vi "Untitled 1.vi"() -> ()   [LabVIEW 2012]
uses:
  Control 1.ctl
panel:
  out "Boolean":bool
  in  "OK Button 7":bool
  in  "CE":bool
  in  "MC":bool
  in  "MR":bool
  in  "MS":bool
  in  "x^2":bool
  in  "1/x":bool
  in  "sqrt":bool
  in  "+/-":bool
  in  "-":bool
  in  "x":bool
  in  "/":bool
  in  "C":bool
  in  ",":bool
  in  "0":bool
  in  "9":bool
  in  "8":bool
  in  "7":bool
  in  "6":bool
  in  "5":bool
  in  "4":bool
  in  "3":bool
  out "екран":string
  in  "=":bool
  in  "+":bool
  in  "2":bool
  in  "1":bool
  in  "stop":bool
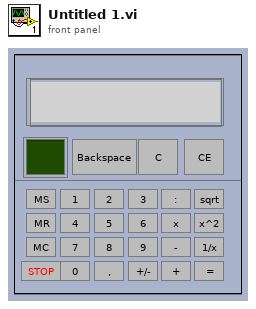
[diagram p1: front panel]
types:
  T1 = typedef "Control 1.ctl" = enum16{"mc", "mr", "ms", "ce", "c", "1/x", "x^2", "sqrt", "+/-", "m", "x", "/", ",", "4", "5", "6", "7", "8", "9", "0", "3", "event", "стоп", "1", "2", "+", "="}
  T2 = cluster{"екран":string, "чистий екран":string, "буфер":string, "Enum":T1, "ms":string, "mr":string}
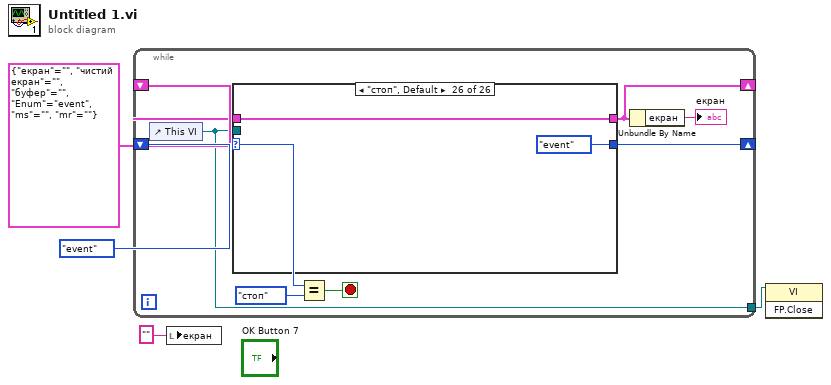
[diagram p0: block diagram]
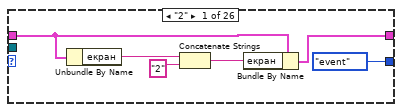
[diagram p2: hidden frame]
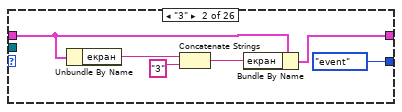
[diagram p3: hidden frame]
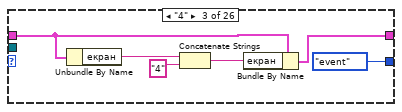
[diagram p4: hidden frame]
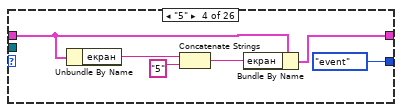
[diagram p5: hidden frame]
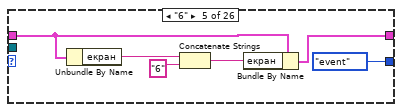
[diagram p6: hidden frame]
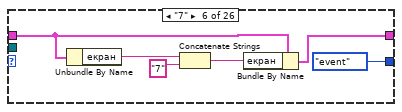
[diagram p7: hidden frame]
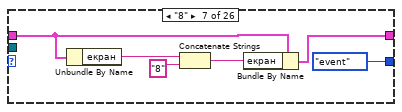
[diagram p8: hidden frame]
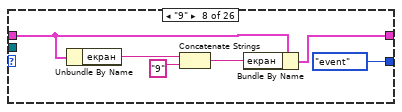
[diagram p9: hidden frame]
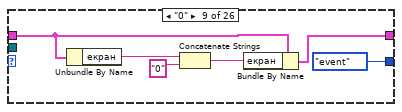
[diagram p10: hidden frame]
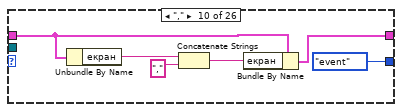
[diagram p11: hidden frame]
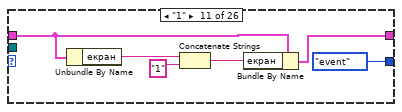
[diagram p12: hidden frame]
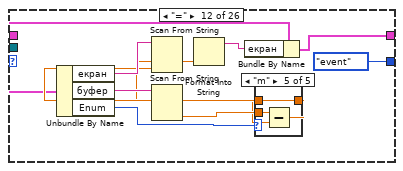
[diagram p13: hidden frame]
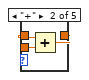
[diagram p15: hidden frame]
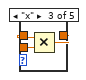
[diagram p16: hidden frame]
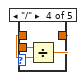
[diagram p17: hidden frame]
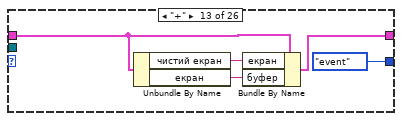
[diagram p18: hidden frame]
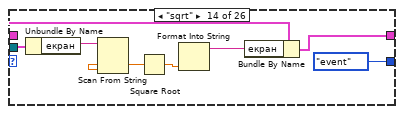
[diagram p19: hidden frame]
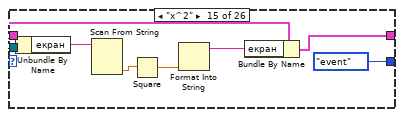
[diagram p20: hidden frame]
diagram:
  n1 = while {
    shift-right: [w12] -> _
    shift-left: Control_1."event" ("Enum") -> [w6]
    shift-right: [w8] -> _
    shift-left: T2 {"екран"="", "чистий екран"="", "буфер"="", "Enum"=enum."event", "ms"="", "mr"=""} -> [w9]
    tunnel: [w5] -> w1
    stop <- w10 stop-if-true
    n2 = control-ref of="This VI"() -> (w5:refnum<vi>)
    n3 = case shown="\"стоп\", Default" w6 {
      tunnel: [Control_1."event" ("Enum") Control_1."event" ("Enum") Control_1."event" ("Enum") Control_1."event" ("Enum") Control_1."event" ("Enum") Control_1."event" ("Enum") Control_1."event" ("Enum") Control_1."event" ("Enum") Control_1."event" ("Enum") Control_1."event" ("Enum") Control_1."event" ("Enum") Control_1."event" ("Enum") Control_1."event" ("Enum") Control_1."event" ("Enum") Control_1."event" ("Enum") Control_1."event" ("Enum") Control_1."event" ("Enum") Control_1."event" ("Enum") Control_1."event" ("Enum") w145 Control_1."event" ("Enum") Control_1."event" ("Enum") Control_1."event" ("Enum") Control_1."event" ("Enum") Control_1."event" ("Enum") Control_1."event" ("Enum")] -> w12
      tunnel: w9 -> [w17 w23 w29 w35 w41 w47 w53 w59 w65 w71 w75 w81 w105 w113 w120 w127 w131 w136 w141 w144 w246 w251 w255 w260 w264 w265]
      tunnel: [w16 w22 w28 w34 w40 w46 w52 w58 w64 w70 w74 w79 w104 w112 w119 w126 w130 w135 w140 w143 _ w250 w252 w258 w261 w265] -> w8
      tunnel: w5 -> [_ _ _ _ _ _ _ _ _ _ _ _ _ _ _ _ _ _ _ _ _ _ _ _ _ _]
      frame "2" {
        n4 = Unbundle By Name(w17) -> ("екран"=w15:string)
        n5 = Concatenate Strings(w15, "2" ("string")) -> (w13:string)
        n6 = Bundle By Name(cluster=w17, "екран"=w13) -> (w16:T2)
      }
      frame "3" {
        n7 = Unbundle By Name(w23) -> ("екран"=w21:string)
        n8 = Concatenate Strings(w21, "3" ("string")) -> (w19:string)
        n9 = Bundle By Name(cluster=w23, "екран"=w19) -> (w22:T2)
      }
      frame "4" {
        n10 = Unbundle By Name(w29) -> ("екран"=w27:string)
        n11 = Concatenate Strings(w27, "4" ("string")) -> (w25:string)
        n12 = Bundle By Name(cluster=w29, "екран"=w25) -> (w28:T2)
      }
      frame "5" {
        n13 = Unbundle By Name(w35) -> ("екран"=w33:string)
        n14 = Concatenate Strings(w33, "5" ("string")) -> (w31:string)
        n15 = Bundle By Name(cluster=w35, "екран"=w31) -> (w34:T2)
      }
      frame "6" {
        n16 = Unbundle By Name(w41) -> ("екран"=w39:string)
        n17 = Concatenate Strings(w39, "6" ("string")) -> (w37:string)
        n18 = Bundle By Name(cluster=w41, "екран"=w37) -> (w40:T2)
      }
      frame "7" {
        n19 = Unbundle By Name(w47) -> ("екран"=w45:string)
        n20 = Concatenate Strings(w45, "7" ("string")) -> (w43:string)
        n21 = Bundle By Name(cluster=w47, "екран"=w43) -> (w46:T2)
      }
      frame "8" {
        n22 = Unbundle By Name(w53) -> ("екран"=w51:string)
        n23 = Concatenate Strings(w51, "8" ("string")) -> (w49:string)
        n24 = Bundle By Name(cluster=w53, "екран"=w49) -> (w52:T2)
      }
      frame "9" {
        n25 = Unbundle By Name(w59) -> ("екран"=w57:string)
        n26 = Concatenate Strings(w57, "9" ("string")) -> (w55:string)
        n27 = Bundle By Name(cluster=w59, "екран"=w55) -> (w58:T2)
      }
      frame "0" {
        n28 = Unbundle By Name(w65) -> ("екран"=w63:string)
        n29 = Concatenate Strings(w63, "0" ("string")) -> (w61:string)
        n30 = Bundle By Name(cluster=w65, "екран"=w61) -> (w64:T2)
      }
      frame "," {
        n31 = Unbundle By Name(w71) -> ("екран"=w69:string)
        n32 = Concatenate Strings(w69, "," ("string")) -> (w67:string)
        n33 = Bundle By Name(cluster=w71, "екран"=w67) -> (w70:T2)
      }
      frame "1" {
        n34 = Unbundle By Name(w75) -> ("екран"=w77:string)
        n35 = Concatenate Strings(w77, "1" ("string")) -> (w73:string)
        n36 = Bundle By Name(cluster=w75, "екран"=w73) -> (w74:T2)
      }
      frame "=" {
        n37 = Unbundle By Name(w81) -> ("екран"=w86:string, "буфер"=w84:string, "Enum"=w87:T1)
        n38 = Scan From String(input string=w86) -> (output 1=w85:dbl)  [unwired: 4 in, 3 out]
        n39 = Scan From String(input string=w84) -> (output 1=w83:dbl)  [unwired: 4 in, 3 out]
        n40 = case shown="\"m\"" w87 {
          tunnel: w85 -> [w89 w92 w94 w97 w99]
          tunnel: w83 -> [_ w91 w95 w96 w100]
          tunnel: [w89 w90 w93 w98 w101] -> w82
          frame "event", Default {
          }
          frame "+" {
            n41 = Add(x=w92, y=w91) -> (x+y=w90:dbl)
          }
          frame "x" {
            n42 = Multiply(x=w94, y=w95) -> (x*y=w93:dbl)
          }
          frame "/" {
            n43 = Divide(x=w96, y=w97) -> (x/y=w98:dbl)
          }
          frame "m" {
            n44 = Subtract(x=w100, y=w99) -> (x-y=w101:dbl)
          }
        }
        n45 = Format Into String(w82) -> (resulting string=w80:string)  [unwired: 3 in, 1 out]
        n46 = Bundle By Name(cluster=w81, "екран"=w80) -> (w79:T2)
      }
      frame "+" {
        n47 = Unbundle By Name(w105) -> ("чистий екран"=w103:string, "екран"=w102:string)
        n48 = Bundle By Name(cluster=w105, "екран"=w103, "буфер"=w102) -> (w104:T2)
      }
      frame "sqrt" {
        n49 = Unbundle By Name(w113) -> ("екран"=w111:string)
        n50 = Scan From String(input string=w111) -> (output 1=w110:dbl)  [unwired: 4 in, 3 out]
        n51 = Square Root(x=w110) -> (sqrt(x)=w109:dbl)
        n52 = Format Into String(w109) -> (resulting string=w108:string)  [unwired: 3 in, 1 out]
        n53 = Bundle By Name(cluster=w113, "екран"=w108) -> (w112:T2)
      }
      frame "x^2" {
        n54 = Unbundle By Name(w120) -> ("екран"=w118:string)
        n55 = Scan From String(input string=w118) -> (output 1=w116:dbl)  [unwired: 4 in, 3 out]
        n56 = Square(x=w116) -> (x^2=w115:dbl)
        n57 = Format Into String(w115) -> (resulting string=w117:string)  [unwired: 3 in, 1 out]
        n58 = Bundle By Name(cluster=w120, "екран"=w117) -> (w119:T2)
      }
      frame "1/x" {
        n59 = Unbundle By Name(w127) -> ("екран"=w124:string)
        n60 = Scan From String(input string=w124) -> (output 1=w123:dbl)  [unwired: 4 in, 3 out]
        n61 = Reciprocal(x=w123) -> (1/x=w122:dbl)
        n62 = Format Into String(w122) -> (resulting string=w125:string)  [unwired: 3 in, 1 out]
        n63 = Bundle By Name(cluster=w127, "екран"=w125) -> (w126:T2)
      }
      frame "/" {
        n64 = Unbundle By Name(w131) -> ("чистий екран"=w129:string, "екран"=w128:string)
        n65 = Bundle By Name(cluster=w131, "екран"=w129, "буфер"=w128) -> (w130:T2)
      }
      frame "m" {
        n66 = Unbundle By Name(w136) -> ("чистий екран"=w134:string, "екран"=w133:string)
        n67 = Bundle By Name(cluster=w136, "екран"=w134, "буфер"=w133) -> (w135:T2)
      }
      frame "x" {
        n68 = Unbundle By Name(w141) -> ("чистий екран"=w139:string, "екран"=w138:string)
        n69 = Bundle By Name(cluster=w141, "екран"=w139, "буфер"=w138) -> (w140:T2)
      }
      frame "event" {
        n70 = event shown="[0] \"stop\": Value Change" {
          selector: _ -> [_ _ _ _ _ _ _ _ _ _ _ _ _ _ _ _ _ _ _ _ _ _ _ _ _ _ _]
          dyn-events: _ -> [_ _ _ _ _ _ _ _ _ _ _ _ _ _ _ _ _ _ _ _ _ _ _ _ _ _ _]
          timeout: _ -> [_ _ _ _ _ _ _ _ _ _ _ _ _ _ _ _ _ _ _ _ _ _ _ _ _ _ _]
          tunnel: [Control_1."стоп" ("Enum") Control_1."event" ("Enum") Control_1."event" ("Enum") w161 Control_1."1" ("Enum") Control_1."2" ("Enum") Control_1."3" ("Enum") Control_1."4" ("Enum") Control_1."5" ("Enum") Control_1."6" ("Enum") Control_1."7" ("Enum") Control_1."8" ("Enum") Control_1."9" ("Enum") Control_1."0" ("Enum") Control_1."," ("Enum") w209 w212 w215 w218 w221 w224 w227 w230 w233 w236 w239 Control_1."=" ("Enum")] -> w145
          tunnel: w144 -> [w146 w151 w154 w160 w187 w189 w191 w193 w195 w197 w199 w201 w203 w205 w207 w211 w213 w216 w220 w223 w226 w229 w232 w235 w238 w240 w242]
          tunnel: [w146 w149 w158 w159 w187 w189 w191 w193 w195 w197 w199 w201 w203 w205 w207 w210 w214 w217 w219 w222 w225 w228 w231 w234 w237 w241 w242] -> w143
          event "stop": Value Change {
            n71 = event-data() -> ()  [unwired: 1 in, 5 out]
          }
          event "C": Value Change {
            n72 = event-data() -> ()  [unwired: 1 in, 5 out]
            n73 = Bundle By Name(cluster=w151, "екран"="") -> (w149:T2)
          }
          event "+/-": Value Change {
            n74 = Unbundle By Name(w154) -> ("екран"=w155:string)
            n75 = event-data() -> ()  [unwired: 1 in, 5 out]
            n76 = Concatenate Strings("-", w155) -> (w153:string)
            n77 = String Subset(string=w153, length (rest)=1 ("length (rest)")) -> ()  [unwired: 1 in, 1 out]
            n78 = Bundle By Name(cluster=w154, "екран"=w153) -> (w158:T2)
          }
          event Menu Selection (User) {
            n79 = event-data() -> ("ItemTag"=w162:string)  [unwired: 1 in, 5 out]
            n80 = case shown="\"корінь\"" w162 {
              tunnel: w160 -> [w165 w168 w171 w174 w177 w180 w183 w186]
              tunnel: [w163 w167 w170 w173 w175 w178 w181 w185] -> w161
              tunnel: [w164 w166 w169 w172 w176 w179 w182 w184] -> w159
              frame "додати", Default {
                w163 = Control_1."+" ("Enum")
                n81 = Bundle By Name(cluster=w165, "Enum"=w163) -> (w164:T2)
              }
              frame "відняти" {
                w167 = Control_1."m" ("Enum")
                n82 = Bundle By Name(cluster=w168, "Enum"=w167) -> (w166:T2)
              }
              frame "поділити" {
                w170 = Control_1."/" ("Enum")
                n83 = Bundle By Name(cluster=w171, "Enum"=w170) -> (w169:T2)
              }
              frame "помножити" {
                w173 = Control_1."x" ("Enum")
                n84 = Bundle By Name(cluster=w174, "Enum"=w173) -> (w172:T2)
              }
              frame "квадрат" {
                w175 = Control_1."x^2" ("Enum")
                n85 = Bundle By Name(cluster=w177, "Enum"=w175) -> (w176:T2)
              }
              frame "1/х" {
                w178 = Control_1."1/x" ("Enum")
                n86 = Bundle By Name(cluster=w180, "Enum"=w178) -> (w179:T2)
              }
              frame "стоп" {
                w181 = Control_1."стоп" ("Enum")
                n87 = Bundle By Name(cluster=w183, "Enum"=w181) -> (w182:T2)
              }
              frame "корінь" {
                w185 = Control_1."sqrt" ("Enum")
                n88 = Bundle By Name(cluster=w186, "Enum"=w185) -> (w184:T2)
              }
            }
          }
          event "1": Value Change {
            n89 = event-data() -> ()  [unwired: 1 in, 5 out]
          }
          event "2": Value Change {
            n90 = event-data() -> ()  [unwired: 1 in, 5 out]
          }
          event "3": Value Change {
            n91 = event-data() -> ()  [unwired: 1 in, 5 out]
          }
          event "4": Value Change {
            n92 = event-data() -> ()  [unwired: 1 in, 5 out]
          }
          event "5": Value Change {
            n93 = event-data() -> ()  [unwired: 1 in, 5 out]
          }
          event "6": Value Change {
            n94 = event-data() -> ()  [unwired: 1 in, 5 out]
          }
          event "7": Value Change {
            n95 = event-data() -> ()  [unwired: 1 in, 5 out]
          }
          event "8": Value Change {
            n96 = event-data() -> ()  [unwired: 1 in, 5 out]
          }
          event "9": Value Change {
            n97 = event-data() -> ()  [unwired: 1 in, 5 out]
          }
          event "0": Value Change {
            n98 = event-data() -> ()  [unwired: 1 in, 5 out]
          }
          event ",": Value Change {
            n99 = event-data() -> ()  [unwired: 1 in, 5 out]
          }
          event "+": Value Change {
            w209 = Control_1."+" ("Enum")
            n100 = event-data() -> ()  [unwired: 1 in, 5 out]
            n101 = Bundle By Name(cluster=w211, "Enum"=w209) -> (w210:T2)
          }
          event "/": Value Change {
            w212 = Control_1."/" ("Enum")
            n102 = event-data() -> ()  [unwired: 1 in, 5 out]
            n103 = Bundle By Name(cluster=w213, "Enum"=w212) -> (w214:T2)
          }
          event "x": Value Change {
            w215 = Control_1."x" ("Enum")
            n104 = event-data() -> ()  [unwired: 1 in, 5 out]
            n105 = Bundle By Name(cluster=w216, "Enum"=w215) -> (w217:T2)
          }
          event "sqrt": Value Change {
            w218 = Control_1."sqrt" ("Enum")
            n106 = event-data() -> ()  [unwired: 1 in, 5 out]
            n107 = Bundle By Name(cluster=w220, "Enum"=w218) -> (w219:T2)
          }
          event "CE": Value Change {
            w221 = Control_1."ce" ("Enum")
            n108 = event-data() -> ()  [unwired: 1 in, 5 out]
            n109 = Bundle By Name(cluster=w223, "Enum"=w221) -> (w222:T2)
          }
          event "x^2": Value Change {
            w224 = Control_1."x^2" ("Enum")
            n110 = event-data() -> ()  [unwired: 1 in, 5 out]
            n111 = Bundle By Name(cluster=w226, "Enum"=w224) -> (w225:T2)
          }
          event "1/x": Value Change {
            w227 = Control_1."1/x" ("Enum")
            n112 = event-data() -> ()  [unwired: 1 in, 5 out]
            n113 = Bundle By Name(cluster=w229, "Enum"=w227) -> (w228:T2)
          }
          event "MS": Value Change {
            w230 = Control_1."ms" ("Enum")
            n114 = event-data() -> ()  [unwired: 1 in, 5 out]
            n115 = Bundle By Name(cluster=w232, "Enum"=w230) -> (w231:T2)
          }
          event "MR": Value Change {
            w233 = Control_1."mr" ("Enum")
            n116 = event-data() -> ()  [unwired: 1 in, 5 out]
            n117 = Bundle By Name(cluster=w235, "Enum"=w233) -> (w234:T2)
          }
          event "MC": Value Change {
            w236 = Control_1."mc" ("Enum")
            n118 = event-data() -> ()  [unwired: 1 in, 5 out]
            n119 = Bundle By Name(cluster=w238, "Enum"=w236) -> (w237:T2)
          }
          event "-": Value Change {
            w239 = Control_1."m" ("Enum")
            n120 = event-data() -> ()  [unwired: 1 in, 5 out]
            n121 = Bundle By Name(cluster=w240, "Enum"=w239) -> (w241:T2)
          }
          event "=": Value Change {
            n122 = event-data() -> ()  [unwired: 1 in, 5 out]
          }
        }
      }
      frame "c" {
        n123 = Unbundle By Name(w246) -> ("чистий екран"=w245:string)
        n124 = Bundle By Name(cluster=w246, "екран"=w245, "буфер"=w245) -> ()  [unwired: 1 out]
      }
      frame "ms" {
        n125 = Unbundle By Name(w251) -> ("екран"=w249:string)
        n126 = Bundle By Name(cluster=w251, "ms"=w249) -> (w250:T2)
        "Boolean" <- TRUE
      }
      frame "mr" {
        n127 = Unbundle By Name(w255) -> ("ms"=w254:string)
        n128 = Bundle By Name(cluster=w255, "екран"=w254) -> (w252:T2)
      }
      frame "mc" {
        n129 = local write "Boolean"(FALSE) -> ()
        n130 = Unbundle By Name(w260) -> ("чистий екран"=w259:string)
        n131 = Bundle By Name(cluster=w260, "ms"=w259) -> (w258:T2)
      }
      frame "ce" {
        n132 = Unbundle By Name(w264) -> ("чистий екран"=w263:string)
        n133 = Bundle By Name(cluster=w264, "екран"=w263) -> (w261:T2)
      }
      frame "стоп", Default {
      }
    }
    n134 = Equal?(x=w6, y=Control_1."стоп" ("Enum")) -> (x = y?=w10:bool)
    n135 = Unbundle By Name(w8) -> ("екран"=→"екран":string)
  }
  n136 = local write "екран"("") -> ()
  n137 = invoke class="VI" method="FP.Close"(reference=w1) -> ()  [unwired: 2 in, 3 out]
